vi "MessagingClassExample.vi"() -> ()   [LabVIEW 2023]
uses:
  Messaging/Messaging.lvclass
  Msg/Msg.Q.DequeueMode.ctl
panel:
  in  "EHL to MHL":string
  in  "Send MHL to EHL":bool
  out "Received from MHL":string
  in  "MHL to EHL":string
  in  "Stop":bool
  out "Received from EHL":string
  in  "Send EHL to MHL":bool
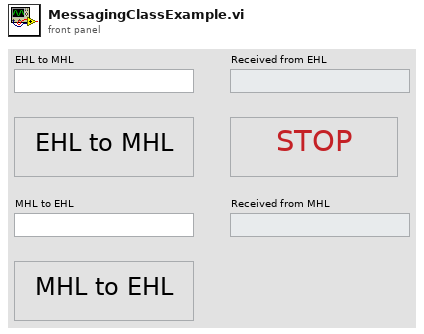
[diagram p1: front panel]
types:
  T1 = typedef "Msg.Event.RegRef.ctl" = refnum<event-registration>
  T2 = typedef "Msg.Q.DequeueMode.ctl" = enum16{"Standard", "Preview"}
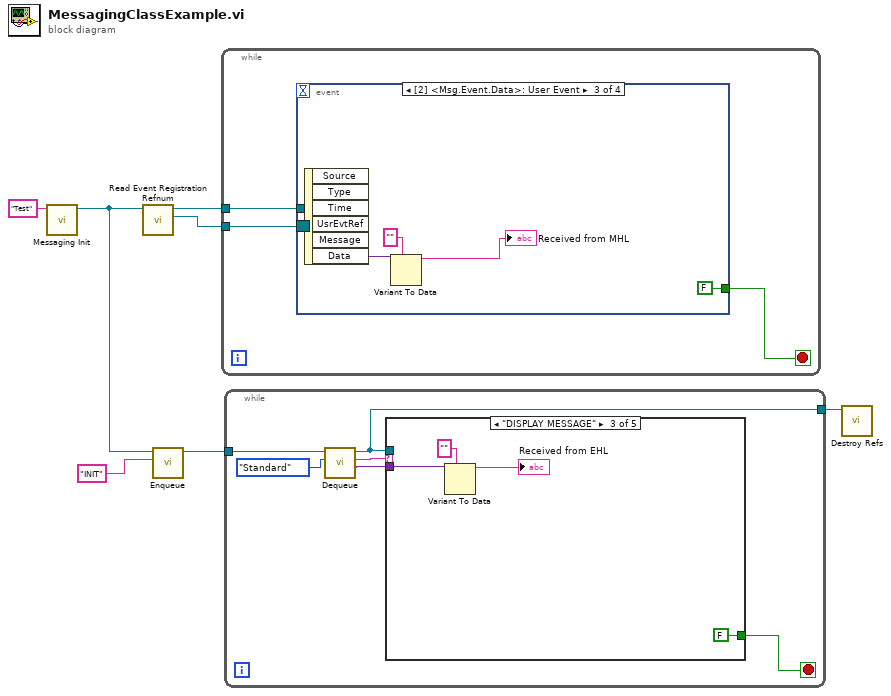
[diagram p0: block diagram]
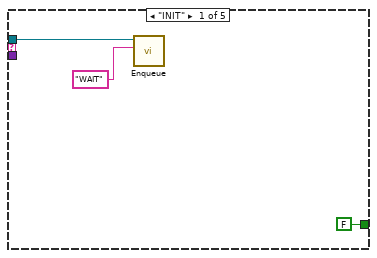
[diagram p2: hidden frame]
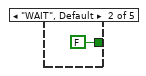
[diagram p3: hidden frame]
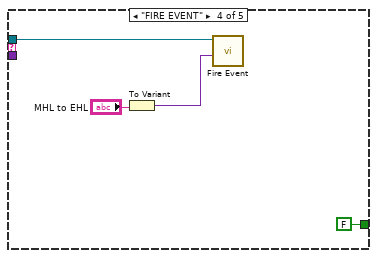
[diagram p4: hidden frame]
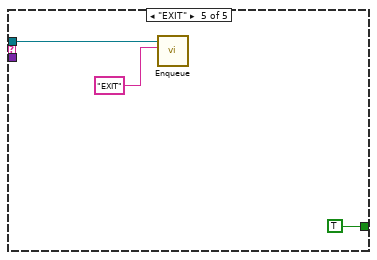
[diagram p5: hidden frame]
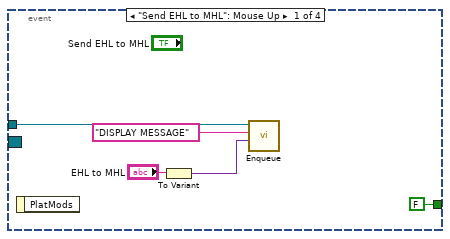
[diagram p6: hidden frame]
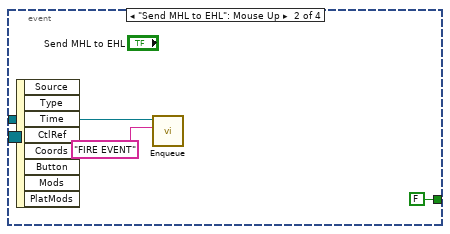
[diagram p7: hidden frame]
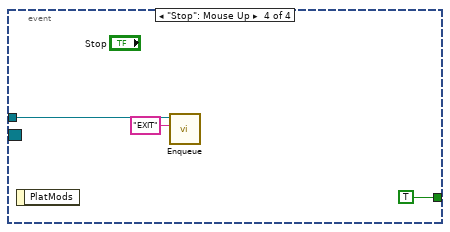
[diagram p8: hidden frame]
diagram:
  n1 = call "Messaging Init.vi"("References Name (in)"="Test" ("Queue Name (in)")) -> ("Messaging out"=w1:refnum<class "Messaging.lvclass">)  [unwired: 8 in, 2 out]
  n2 = call-dynamic "Read Event Registration Refnum.vi"("Messaging in"=w1) -> ("Event Registration Refnum"=w5:T1, "Messaging out"=w4:refnum<class "Messaging.lvclass">)  [unwired: 8 in, 1 out]
  n3 = call "Enqueue.vi"("Message"="INIT", "Messaging in"=w1) -> ("Messaging out"=w6:refnum<class "Messaging.lvclass">)  [unwired: 8 in, 1 out]
  n4 = while {
    tunnel: w4 -> [w10]
    tunnel: w5 -> [w9]
    stop <- w8 stop-if-true
    n5 = event shown="[2] <Msg.Event.Data>: User Event" {
      selector: w9 -> [_ _ _ _]
      dyn-events: _ -> [_ _ _ _]
      timeout: _ -> [_ _ _ _]
      tunnel: w10 -> [w15 w18 _ w25]
      tunnel: [FALSE FALSE FALSE TRUE] -> w8
      event "Send EHL to MHL": Mouse Up {
        n6 = event-data() -> ()  [unwired: 1 in, 1 out]
        n7 = To Variant(anything="EHL to MHL") -> (Variant=w12:variant)
        n8 = call "Enqueue.vi"("Data"=w12, "Message"="DISPLAY MESSAGE", "Messaging in"=w15) -> ()  [unwired: 7 in, 2 out]
      }
      event "Send MHL to EHL": Mouse Up {
        n9 = event-data() -> ()  [unwired: 1 in, 8 out]
        n10 = call "Enqueue.vi"("Message"="FIRE EVENT", "Messaging in"=w18) -> ()  [unwired: 8 in, 2 out]
      }
      event User Event {
        n11 = event-data() -> ("Data"=w22:variant)  [unwired: 1 in, 5 out]
        n12 = Variant To Data(type="", Variant=w22) -> (data=→"Received from MHL":string)  [unwired: 1 in, 1 out]
      }
      event "Stop": Mouse Up {
        n13 = event-data() -> ()  [unwired: 1 in, 1 out]
        n14 = call "Enqueue.vi"("Message"="EXIT", "Messaging in"=w25) -> ()  [unwired: 8 in, 2 out]
      }
    }
  }
  n15 = while {
    tunnel: w6 -> [w29]
    tunnel: [w28] -> w2
    stop <- w31 stop-if-true
    n16 = call "Dequeue.vi"("Dequeue Mode"=Msg.Q.DequeueMode."Standard", "Messaging in"=w29) -> ("Data"=w26:variant, "Message"=w27:string, "Messaging out"=w28:refnum<class "Messaging.lvclass">)  [unwired: 6 in, 1 out]
    n17 = case shown="\"DISPLAY MESSAGE\"" w27 {
      tunnel: w28 -> [w32 _ _ w40 w44]
      tunnel: w26 -> [_ _ w39 _ _]
      tunnel: [FALSE FALSE FALSE FALSE TRUE] -> w31
      frame "INIT" {
        n18 = call "Enqueue.vi"("Message"="WAIT", "Messaging in"=w32) -> ()  [unwired: 8 in, 2 out]
      }
      frame "WAIT", Default {
      }
      frame "DISPLAY MESSAGE" {
        n19 = Variant To Data(type="", Variant=w39) -> (data=→"Received from EHL":string)  [unwired: 1 in, 1 out]
      }
      frame "FIRE EVENT" {
        n20 = To Variant(anything="MHL to EHL") -> (Variant=w41:variant)
        n21 = call "Fire Event.vi"("Data"=w41, "Messaging in"=w40) -> ()  [unwired: 8 in, 2 out]
      }
      frame "EXIT" {
        n22 = call "Enqueue.vi"("Message"="EXIT", "Messaging in"=w44) -> ()  [unwired: 8 in, 2 out]
      }
    }
  }
  n23 = call "Destroy Refs.vi"("Messaging in"=w2) -> ()  [unwired: 10 in, 1 out]
